vi "Message with Response.vi"(6 "Timeout in ms (-1)":i32=-1, 8 "error in (no error)":errorcluster, 9 "Data":variant, 10 "Command":string, 11 "MessageEvent":refnum<user-event>) -> (0 "error out":errorcluster, 3 "Response":variant)   [LabVIEW 2019, in "SLL Message.lvlib"]
uses:
  SLL Message.lvlib
  Typedefs/Message.ctl
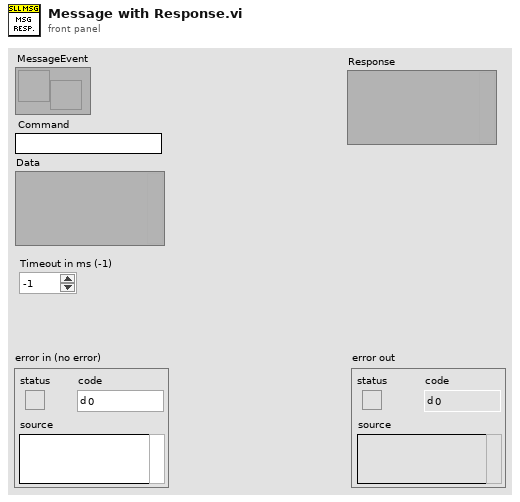
[diagram p1: front panel]
types:
  T1 = typedef "SLL Message.lvlib/Message.ctl" = cluster{"Command":string, "Data":variant, "Fetch Response?":bool, "Response":refnum<notifier>}
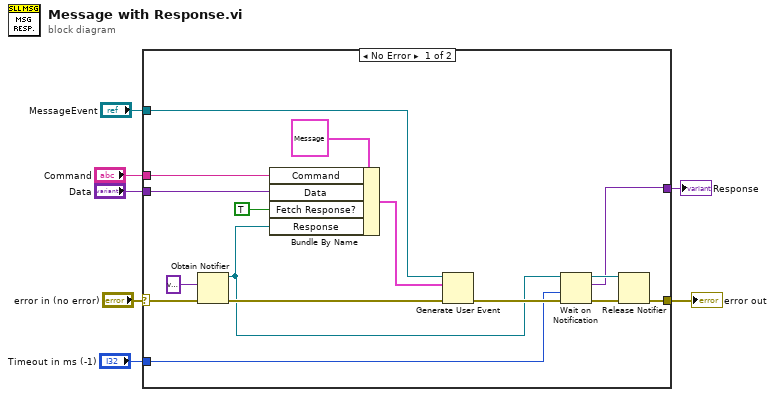
[diagram p0: block diagram]
diagram:
  n1 = case shown="No Error" "error in (no error)" {
    selector: "error in (no error)" -> [w15 w24]
    tunnel: [w10 w24] -> w6
    tunnel: "MessageEvent" -> [w22 _]
    tunnel: "Command" -> [w19 _]
    tunnel: "Data" -> [w18 _]
    tunnel: "Timeout in ms (-1)" -> [w11 _]
    tunnel: [w8 _] -> w1
    frame No Error {
      n2 = Obtain Notifier(notification data type=variant ("element data type"), error in (no error)=w15) -> (notifier out=w12:refnum<notifier>, error out=w14:errorcluster)  [unwired: 2 in, 1 out]
      n3 = Bundle By Name(cluster=T1 {"Command"="", "Data"=variant, "Fetch Response?"=FALSE, "Response"=refnum} ("event data"), "Command"=w19, "Data"=w18, "Fetch Response?"=TRUE, "Response"=w12) -> (w20:T1)
      n4 = Generate User Event(user event=w22, event data cluster=w20, error in=w14) -> (error out=w23:errorcluster)  [unwired: 1 in, 1 out]
      n5 = Wait on Notification(notifier=w12, timeout in ms (-1)=w11, error in (no error)=w23) -> (notifier out=w9:refnum<notifier>, notification=w8:variant, error out=w13:errorcluster)  [unwired: 1 in, 1 out]
      n6 = Release Notifier(notifier=w9, error in (no error)=w13) -> (error out=w10:errorcluster)  [unwired: 1 in, 2 out]
    }
    frame Error {
    }
  }
  "error out" <- w6
  "Response" <- w1
